vi "IMGAutoRotation.vi"(4 "OutputFiles":path, 6 "Threads":i32=4, 8 "error in (no error)":errorcluster caption="错误输入（无错误）", 11 "EPUB 输入":refnum<class "EPUB.lvclass">) -> (0 "error out":errorcluster caption="错误输出", 3 "EPUB 输出":refnum<class "EPUB.lvclass">)   [LabVIEW 2016, in "EPUB.lvclass"]
uses:
  EPUB.lvclass
  EPUB.lvclass/EPUB.ctl
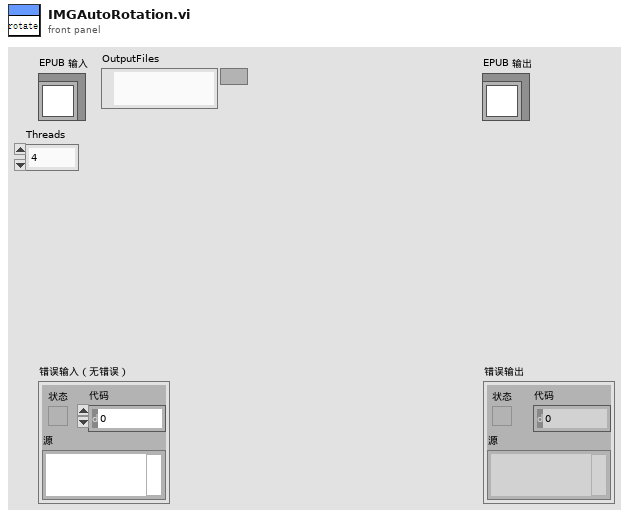
[diagram p1: front panel]
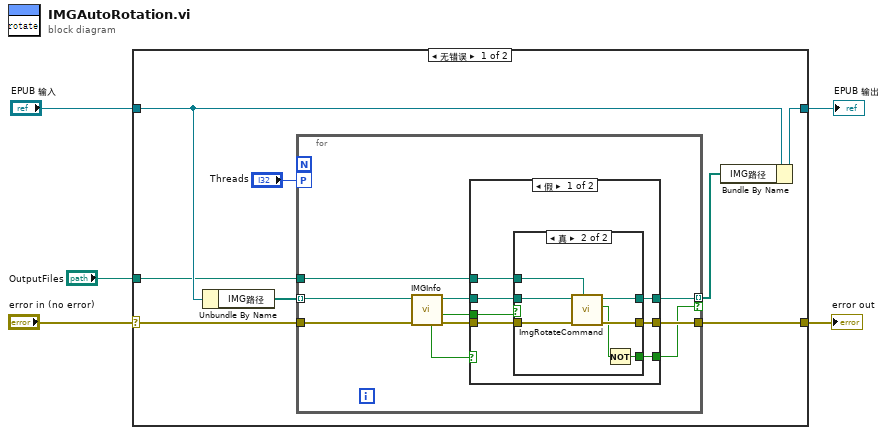
[diagram p0: block diagram]
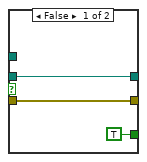
[diagram p2: hidden frame]
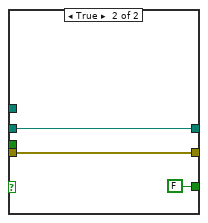
[diagram p3: hidden frame]
diagram:
  n1 = case shown="无错误" "error in (no error)" {
    selector: "error in (no error)" -> [w10 w45]
    tunnel: [w9 w45] -> w4
    tunnel: [w8 w44] -> w2
    tunnel: "EPUB 输入" -> [w13 w44]
    tunnel: "OutputFiles" -> [w6 _]
    frame No Error {
      n2 = Unbundle By Name(w13) -> ("IMG路径"=w12:path[])
      n3 = for {
        tunnel: w12 -> [w15] mode=indexing
        workers-P: "Threads" -> [_]
        tunnel: w10 -> [w21]
        tunnel: [w19] -> w9
        tunnel: [w17] -> w7 mode=indexing if=w16
        tunnel: w6 -> [w14]
        n4 = call "IMGInfo.vi"("Error in"=w21, "ImgPath"=w15) -> ("Error out"=w23:errorcluster, "Landscape"=w20:bool, "ImgPath out"=w22:path, "error"=w18:bool)  [unwired: 5 in, 1 out]
        n5 = case shown="假" w18 {
          tunnel: w23 -> [w30 w43]
          tunnel: w22 -> [w29 w42]
          tunnel: w20 -> [w28 _]
          tunnel: [w27 w43] -> w19
          tunnel: [w25 FALSE] -> w16
          tunnel: [w26 w42] -> w17
          tunnel: w14 -> [w24 _]
          frame False {
            n6 = case shown="真" w28 {
              tunnel: w30 -> [w33 w40]
              tunnel: w29 -> [w32 w39]
              tunnel: [w33 w38] -> w27
              tunnel: [w32 w37] -> w26
              tunnel: [TRUE w35] -> w25
              tunnel: w24 -> [_ w34]
              frame False {
              }
              frame True {
                n7 = call "ImgRotateCommand.vi"("OutputFiles"=w34, "Error in"=w40, "ImgPath"=w39) -> ("Error out"=w38:errorcluster, "error"=w36:bool, "ImgPath out"=w37:path)  [unwired: 6 in]
                n8 = Not(x=w36) -> (.not. x?=w35:bool)
              }
            }
          }
          frame True {
          }
        }
      }
      n9 = Bundle By Name(cluster=w13, "IMG路径"=w7) -> (w8:refnum<class "EPUB.lvclass">)
    }
    frame Error {
    }
  }
  "error out" <- w4
  "EPUB 输出" <- w2
